vi "Get Cards Data.vi"(8 "error in":errorcluster caption="Error In (no error)") -> (0 "error out":errorcluster caption="Error Out", 3 "Cards":T1[](array[typedef]))   [LabVIEW 2016]
uses:
  DAQ-Config/Controls/PSCHN_Card Para.ctl
  DAQ-Config/Controls/PSCHN_Channel Para.ctl
  <vilib>/Pansino Software/LabVIEW Architecture/Queue Management/PSARC_Queue Create_Single.vi
  <vilib>/Pansino Software/LabVIEW Architecture/Queue Management/PSARC_Queue Insert Element.vi
  <vilib>/Pansino Software/LabVIEW Architecture/Queue Management/PSARC_Queue Remove Element.vi
  <vilib>/Pansino Software/LabVIEW Architecture/Queue Management/PSARC_Queue Destroy_Single.vi
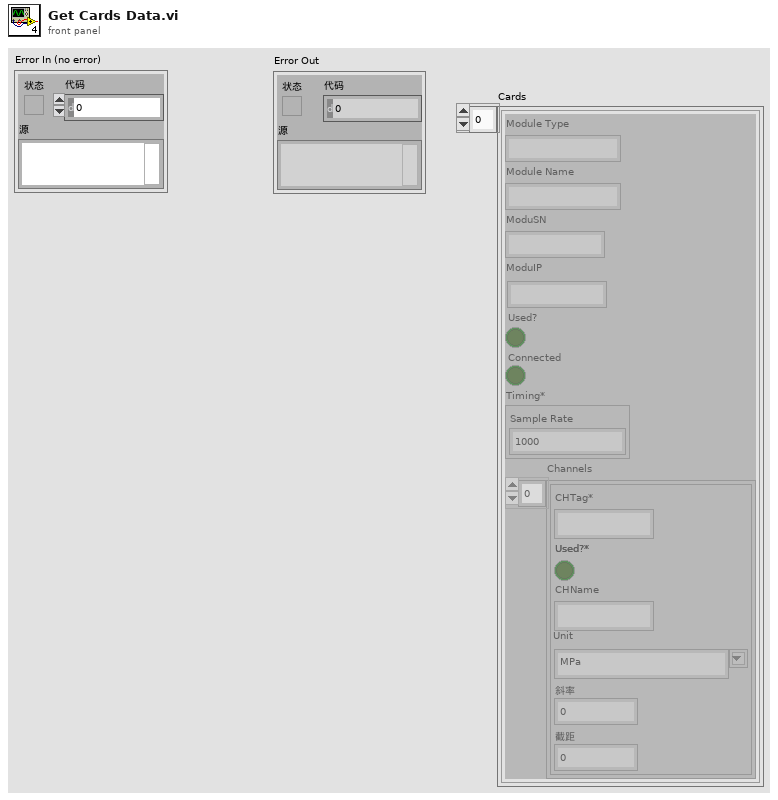
[diagram p1: front panel]
types:
  T1 = typedef "PSCHN_Card Para.ctl" = cluster{"Module Type":string, "Module Name":string, "ModuSN":string, "ModuIP":string, "Used?":bool, "Connected":bool, "Timing*":cluster{"Sample Rate":dbl}, "Channels":T2[]}
  T2 = typedef "PSCHN_Channel Para.ctl" = cluster{"CHTag*":string, "Used?*":bool, "CHName":string, "Unit":string, "斜率":dbl, "截距":dbl}
  T3 = cluster{"Main Queue":string, "DAQ Queue":string, "ANA Queue":string, "CUI Queue":string, "Q-FocusList":string, "Q-Toolbar":string, "Q-Config":string}
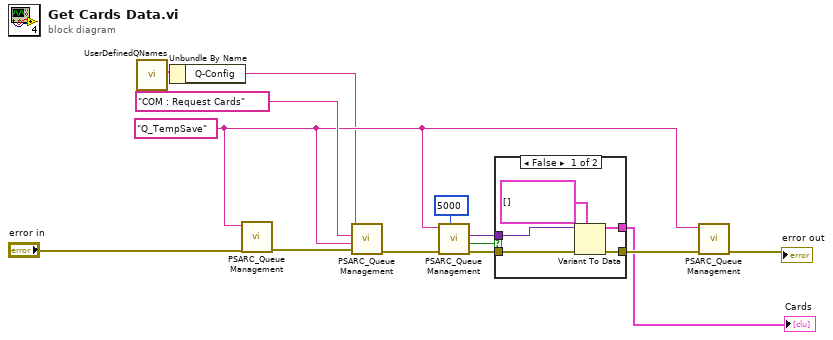
[diagram p0: block diagram]
diagram:
  w10 = "Q_TempSave" ("Queue Name")
  n1 = call "UserDefinedQNames.vi"() -> ("All Queues"=w2:T3)  [unwired: 11 in]
  n2 = Unbundle By Name(w2) -> ("Q-Config"=w1:string)
  n3 = call-poly <vilib>:"PSARC_Queue Management.vi"("error in (no error)"="error in", "Queue Name"=w10) -> ("error out"=w14:errorcluster)  [unwired: 8 in, 1 out]
  n4 = call-poly <vilib>:"PSARC_Queue Management.vi"("error in (no error)"=w14, "Data"=w10, "Event"="COM : Request Cards", "Queue Name(unamed)"=w1) -> ("error out"=w12:errorcluster)  [unwired: 6 in, 1 out]
  n5 = call-poly <vilib>:"PSARC_Queue Management.vi"("Time out(-1)_queue out"=5000, "error in (no error)"=w12, "Queue Name(unamed)"=w10) -> ("error out"=w8:errorcluster, "timed out"=w6:bool, "Data"=w5:variant)  [unwired: 5 in, 1 out]
  n6 = case shown="False" w6 {
    tunnel: w8 -> [w19 w20]
    tunnel: [w18 w20] -> w7
    tunnel: w5 -> [w17 _]
    tunnel: [w16 _] -> w3
    frame False {
      n7 = Variant To Data(error in=w19, type=T1[] [] ("Gen Cards-1"), Variant=w17) -> (data=w16:T1[], error out=w18:errorcluster)
    }
    frame True {
    }
  }
  "Cards" <- w3
  n8 = call-poly <vilib>:"PSARC_Queue Management.vi"("error in (no error)"=w7, "Queue Name(unamed)"=w10) -> ("error out"=→"error out":errorcluster)  [unwired: 7 in, 2 out]
